vi "_Build Exp Parameters.vi"(8 "error in (no error)":errorcluster, 11 "Server Method":T7 {"Expt"."Mass Range"."Res" items=["High/High", "Medium/Medium", "Low/Low", "High/Medium", "High/Low", "Medium/High", "Medium/Low", "Low/High", "Low/Medium"]}) -> (0 "error out":errorcluster, 3 "Exp Parameters":T1 {"Expt"."Mass Range"."Resolution Type" items=["High/High", "Medium/Medium", "Low/Low", "High/Medium", "High/Low", "Medium/High", "Medium/Low", "Low/High", "Low/Medium"]})   [LabVIEW 2015]
uses:
  Type/_Server Method.ctl
  Type/_XML Expt.ctl
  Type/_XML Lens.ctl
  Type/_Mass Range Property.ctl
  Type/_Mass Range Parameters.ctl
  Type/_RT Res Type.ctl
  Type/_RT Active Ch.ctl
  Type/_RT Parameter.ctl
  Type/_RT Expt.ctl
  Type/_Run Mode.ctl
  Type/_RT Mass Range.ctl
panel:
  out "Scans":i32=5
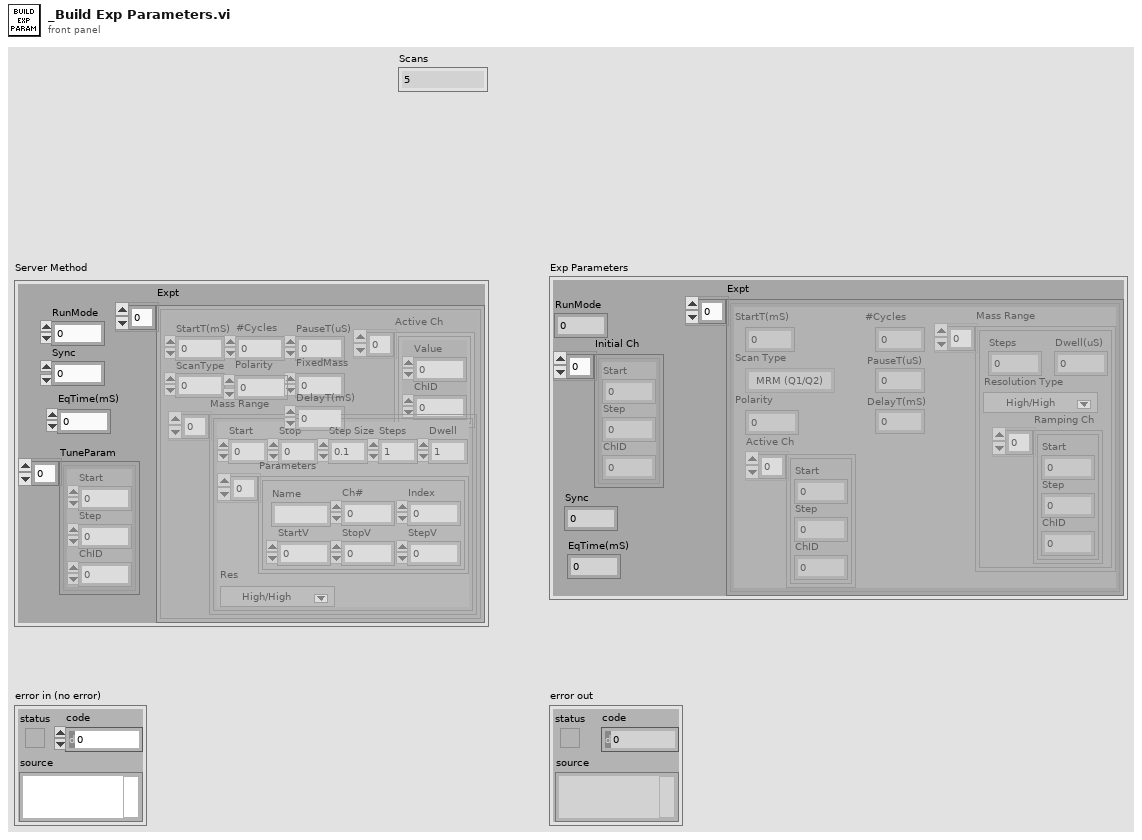
[diagram p1: front panel]
types:
  T1 = typedef "_RT Parameter.ctl" = cluster{"RunMode":i32, "Initial Ch":T2[], "Sync":u8, "Expt":T3[], "EqTime(mS)":i32}
  T2 = typedef "_RT Active Ch.ctl" = cluster{"Start":i32, "Step":i32, "ChID":i32}
  T3 = typedef "_RT Expt.ctl" = cluster{"StartT(mS)":i32, "#Cycles":i32, "Scan Type":T4, "PauseT(uS)":i32, "Polarity":u8, "DelayT(mS)":i32, "Active Ch":T2[], "Mass Range":T5[]}
  T4 = typedef "_Run Mode.ctl" = enum16{"MRM (Q1/Q2)", "Q1 Scan", "Q1 SRM", "Q2 Scan", "Q2 SRM", "Product Scan", "Precursor Scan", "Neutral Loss", "Neutral Gain"}
  T5 = typedef "_RT Mass Range.ctl" = cluster{"Steps":i32, "Dwell(uS)":i32, "Resolution Type":T6, "Ramping Ch":T2[]}
  T6 = typedef "_RT Res Type.ctl" = u16
  T7 = typedef "_Server Method.ctl" = cluster{"RunMode":i32, "Sync":u8, "Expt":T8[], "EqTime(mS)":i32, "TuneParam":T2[]}
  T8 = typedef "_XML Expt.ctl" = cluster{"StartT(mS)":i32, "#Cycles":i32, "PauseT(uS)":i32, "ScanType":i32, "Polarity":u8, "FixedMass":dbl, "DelayT(mS)":i32, "Active Ch":T9[], "Mass Range":T10[]}
  T9 = typedef "_XML Lens.ctl" = cluster{"Value":dbl, "ChID":u8}
  T10 = typedef "_Mass Range Property.ctl" = cluster{"Start":dbl, "Stop":dbl, "Step Size":dbl, "Steps":i32, "Dwell":dbl, "Parameters":T11[], "Res":T6}
  T11 = typedef "_Mass Range Parameters.ctl" = cluster{"Name":string, "Ch#":u8, "StartV":dbl, "StopV":dbl, "StepV":dbl, "Index":u8}
  T12 = typedef "_RT Configuration 2.ctl" = cluster{"Name":string, "Ch#":u8, "Min":dbl, "Max":dbl, "Def+":dbl, "Def-":dbl, "Offset":dbl, "Slope":dbl, "Type":u8, "Description":string, "SettleT":dbl}
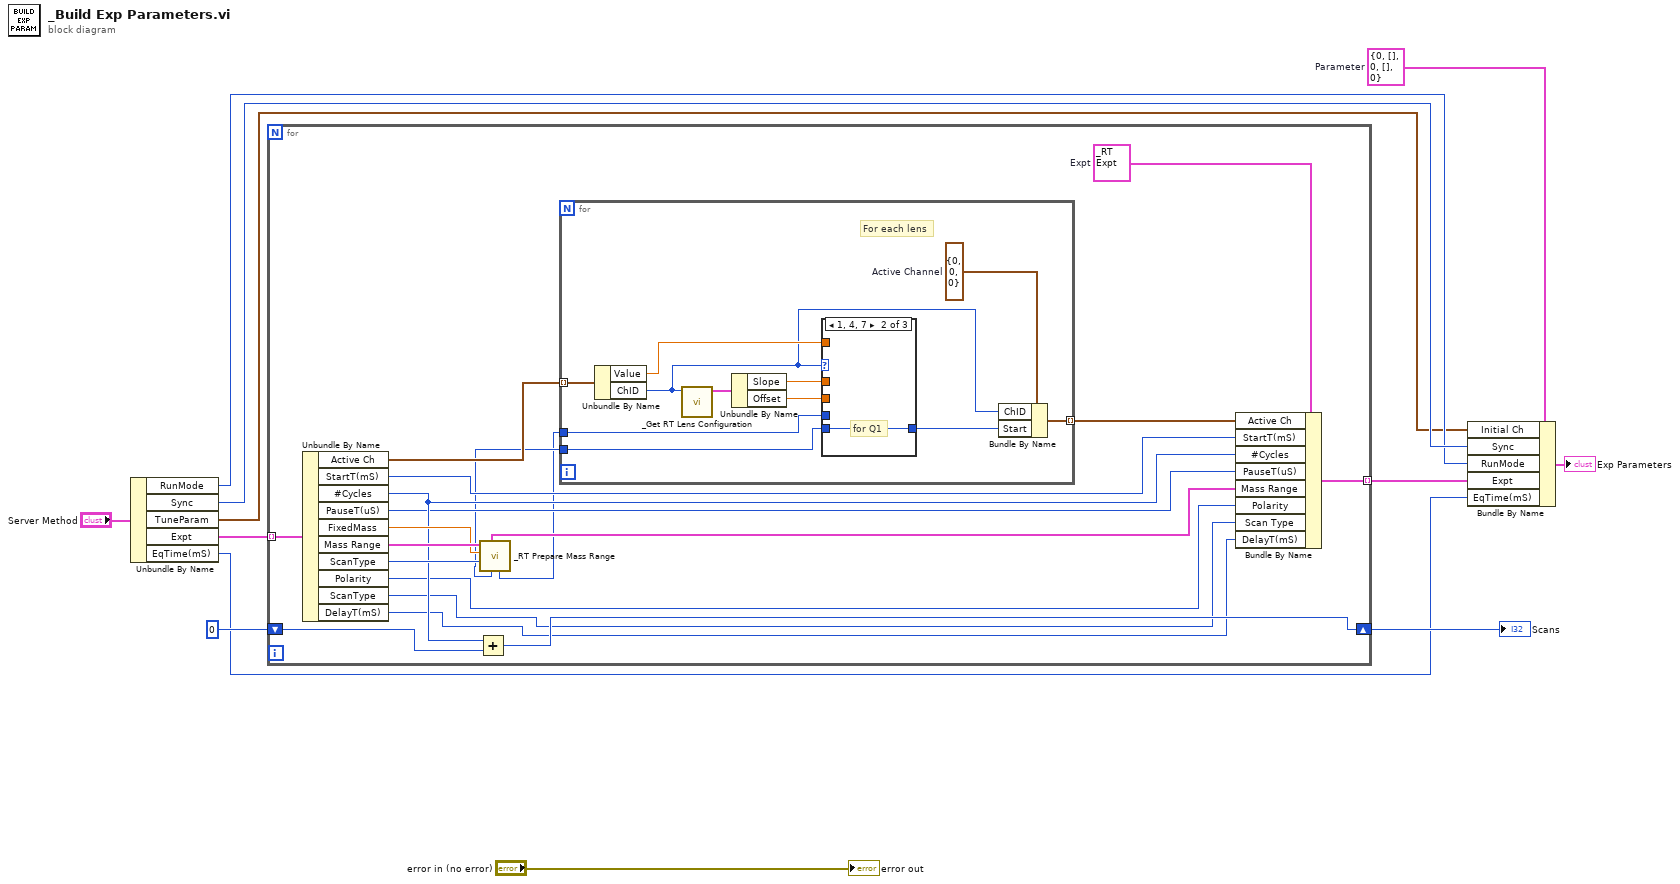
[diagram p0: block diagram]
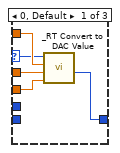
[diagram p2: hidden frame]
diagram:
  w9 = T1 {"RunMode"=0, "Initial Ch"=[], "Sync"=0, "Expt"=[], "EqTime(mS)"=0}  # Parameter
  n1 = Unbundle By Name("Server Method") -> ("RunMode"=w5:i32, "Sync"=w6:u8, "TuneParam"=w4:T2[], "Expt"=w7:T8[], "EqTime(mS)"=w3:i32)
  n2 = for {
    tunnel: w7 -> [w31] mode=indexing
    shift-right: [w26] -> w11
    shift-left: 0 ("index") -> [w27]
    tunnel: [w17] -> w10 mode=indexing
    w13 = T3 {"StartT(mS)"=0, "#Cycles"=1, "Scan Type"=enum."MRM (Q1/Q2)", "PauseT(uS)"=0, "Polarity"=0, "DelayT(mS)"=0, "Active Ch"=[], "Mass Range"=[]}  # Expt
    n3 = Unbundle By Name(w31) -> ("Active Ch"=w21:T9[], "StartT(mS)"=w23:i32, "#Cycles"=w24:i32, "PauseT(uS)"=w22:i32, "FixedMass"=w29:dbl, "Mass Range"=w30:T10[], "ScanType"=w28:i32, "Polarity"=w16:u8, "ScanType"=w15:i32, "DelayT(mS)"=w14:i32)
    n4 = Add(x=w24, y=w27) -> (x+y=w26:i32)
    n5 = call "_RT Prepare Mass Range.vi"("Run Mode"=w28, "Fixed Mass (amu)"=w29, "GUI Mass Ranges"=w30) -> ("Init Q2 Mass"=w18:i32, "Init Q1 Mass"=w19:i32, "RT Mass Ranges"=w25:T5[])  [unwired: 2 in, 4 out]
    n6 = for {
      tunnel: [w38] -> w20 mode=indexing
      tunnel: w21 -> [w37] mode=indexing
      tunnel: w19 -> [w33]
      tunnel: w18 -> [w32]
      w40 = T2 {"Start"=0, "Step"=0, "ChID"=0}  # Active Channel
      # "For each lens"
      n7 = Unbundle By Name(w37) -> ("Value"=w36:dbl, "ChID"=w35:u8)
      n8 = call "_Get RT Lens Configuration.vi"("Channel #"=w35) -> ("Lens Configuration"=w34:T12)  [unwired: 5 in, 1 out]
      n9 = Unbundle By Name(w34) -> ("Slope"=w42:dbl, "Offset"=w41:dbl)
      n10 = case shown="1, 4, 7" w35 {
        selector: w35 -> [w43 _ _]
        tunnel: w36 -> [w47 _ _]
        tunnel: w42 -> [w46 _ _]
        tunnel: w41 -> [w45 _ _]
        tunnel: [w44 w48 w49] -> w39
        tunnel: w33 -> [_ w48 _]
        tunnel: w32 -> [_ _ w49]
        frame 0, Default {
          n11 = call "_RT Convert to DAC Value.vi"("Offset"=w45, "Slop"=w46, "Number"=w47, "Channel"=w43) -> ("DAC Value"=w44:i32)  [unwired: 2 in, 5 out]
        }
        frame 1, 4, 7 {
          # "for Q1"
        }
        frame 2, 5, 9 {
          # "for Q3"
        }
      }
      n12 = Bundle By Name(cluster=w40, "ChID"=w35, "Start"=w39) -> (w38:T2)
    }
    n13 = Bundle By Name(cluster=w13, "Active Ch"=w20, "StartT(mS)"=w23, "#Cycles"=w24, "PauseT(uS)"=w22, "Mass Range"=w25, "Polarity"=w16, "Scan Type"=w15, "DelayT(mS)"=w14) -> (w17:T3)
  }
  "Scans" <- w11
  n14 = Bundle By Name(cluster=w9, "Initial Ch"=w4, "Sync"=w6, "RunMode"=w5, "Expt"=w10, "EqTime(mS)"=w3) -> (→"Exp Parameters":T1)
  "error out" <- "error in (no error)"
